vi "LWXPS_PositionerCorrectorP2IDFFAccelerationGet.vi"(0 "XPS Reference IN":refnum<k24>, 2 "Positioner Name":string, 7 "LabVIEW error IN":errorcluster) -> (9 "LabVIEW error OUT":errorcluster, 10 "XPS Reference OUT":refnum<k24>, 11 "XPS Error String":string, 12 "Returned error code":i32, 13 "Setpoint Position Delay":dbl, 14 "Closed Loop Status":bool, 15 "Feed Forward Jerk":dbl, 16 "Proportional gain":dbl, 17 "Feed Forward Acceleration":dbl, 18 "Integral gain":dbl, 19 "Form coefficient":dbl, 20 "Integral gain 2":dbl, 21 "Derivative gain":dbl, 22 "Integral saturation value":dbl, 23 "Integration time":dbl, 24 "Derivative Filter Cut Off Frequency":dbl, 25 "Proportional gain multiplier":dbl, 26 "Integral gain multiplier":dbl, 27 "Derivative gain multiplier":dbl)   [LabVIEW 2014]
uses:
  D:/XPSQ8_LabView_Library/Development/Source/Dll/Newport.XPS.CommandInterface.dll
  Dll/Newport.XPS.CommandInterface.dll
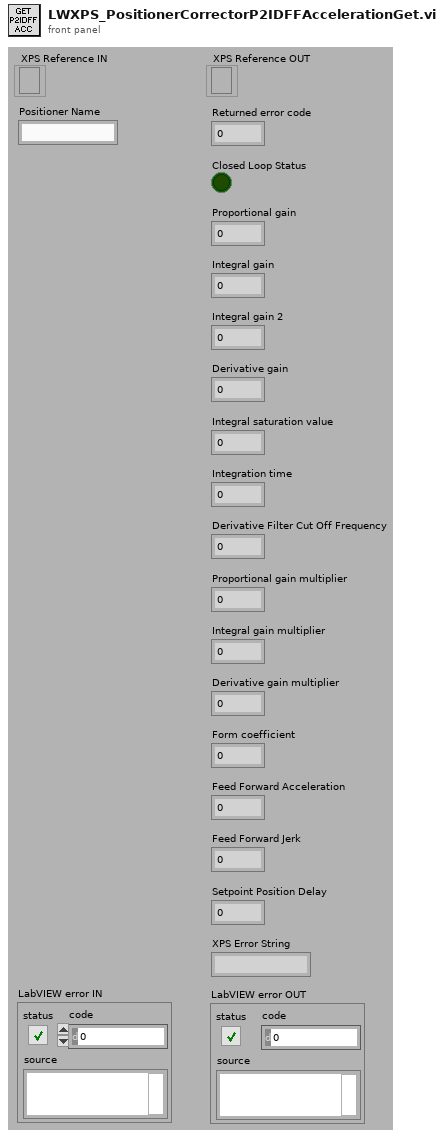
[diagram p1: front panel]
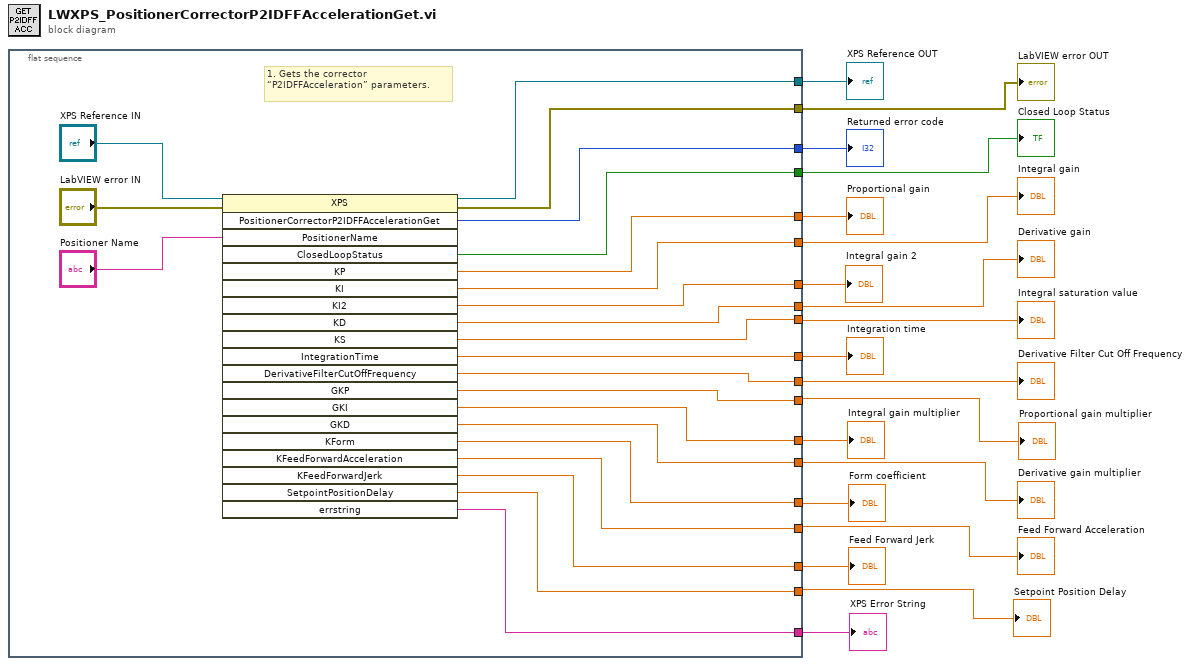
[diagram p0: block diagram]
diagram:
  n1 = flat-sequence {
    tunnel: [w39] -> w10
    tunnel: [w33] -> w19
    tunnel: [w40] -> w18
    tunnel: [w36] -> w17
    tunnel: [w35] -> w1
    tunnel: [w34] -> w16
    tunnel: [w20] -> w15
    tunnel: [w28] -> w14
    tunnel: [w32] -> w11
    tunnel: [w31] -> w13
    tunnel: [w30] -> w12
    tunnel: [w29] -> w3
    tunnel: [w27] -> w9
    tunnel: [w26] -> w8
    tunnel: [w21] -> w7
    tunnel: [w22] -> w6
    tunnel: [w25] -> w5
    tunnel: [w24] -> w2
    tunnel: [w23] -> w4
    frame #0 {
      # "1. Gets the corrector “P2IDFFAcceleration” parameters."
      n2 = invoke class="XPS" method="PositionerCorrectorP2IDFFAccelerationGet"(reference="XPS Reference IN", error in="LabVIEW error IN", "PositionerName"="Positioner Name") -> (reference out=w39:refnum<k24>, error out=w33:errorcluster, "PositionerCorrectorP2IDFFAccelerationGet"=w40:i32, "ClosedLoopStatus"=w32:bool, "KP"=w36:dbl, "KI"=w35:dbl, "KI2"=w34:dbl, "KD"=w20:dbl, "KS"=w28:dbl, "IntegrationTime"=w31:dbl, "DerivativeFilterCutOffFrequency"=w30:dbl, "GKP"=w29:dbl, "GKI"=w27:dbl, "GKD"=w26:dbl, "KForm"=w21:dbl, "KFeedForwardAcceleration"=w22:dbl, "KFeedForwardJerk"=w25:dbl, "SetpointPositionDelay"=w24:dbl, "errstring"=w23:string)  [unwired: 17 in, 1 out]
    }
  }
  "XPS Error String" <- w4
  "XPS Reference OUT" <- w10
  "LabVIEW error OUT" <- w19
  "Returned error code" <- w18
  "Proportional gain" <- w17
  "Integral gain" <- w1
  "Integral gain 2" <- w16
  "Derivative gain" <- w15
  "Integral saturation value" <- w14
  "Integration time" <- w13
  "Derivative Filter Cut Off Frequency" <- w12
  "Closed Loop Status" <- w11
  "Integral gain multiplier" <- w9
  "Derivative gain multiplier" <- w8
  "Form coefficient" <- w7
  "Feed Forward Acceleration" <- w6
  "Feed Forward Jerk" <- w5
  "Setpoint Position Delay" <- w2
  "Proportional gain multiplier" <- w3
